vi "AccelerationAttemptLEDWinker.vi"(6 "inputError":errorcluster, 8 "StateValue":T1, 9 "CurrentEntry":string, 10 "EventProgressDataInput":string[][](array[string]), 11 "inputRefOfLED":refnum<vi>[](array[refnum])) -> (4 "outputError":errorcluster)   [LabVIEW 2020]
uses:
  Control/AccelerationState.ctl
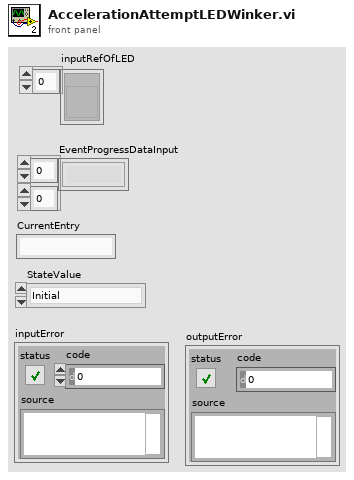
[diagram p1: front panel]
types:
  T1 = typedef "AccelerationState.ctl" = enum16{"Initial", "InputInfomation", "Ready", "Running", "FinshRunning", "LogRecord", "HardwareRelease", "WaittingforNext", "ProgramStop"}
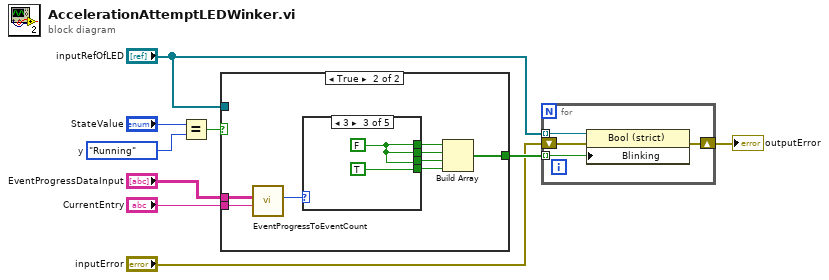
[diagram p0: block diagram]
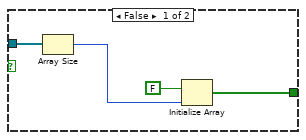
[diagram p2: hidden frame]
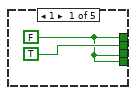
[diagram p3: hidden frame]
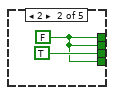
[diagram p4: hidden frame]
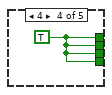
[diagram p5: hidden frame]
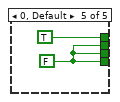
[diagram p6: hidden frame]
diagram:
  w1 = AccelerationState."Running"  # y
  n1 = Equal?(x="StateValue", y=w1) -> (x = y?=w2:bool)
  n2 = case shown="True" w2 {
    tunnel: "EventProgressDataInput" -> [_ w20]
    tunnel: "CurrentEntry" -> [_ w19]
    tunnel: [w9 w18] -> w6
    tunnel: "inputRefOfLED" -> [w12 _]
    frame False {
      n3 = Array Size(array=w12) -> (size(s)=w11:i32)
      n4 = Initialize Array "Initialize Array"(FALSE, w11) -> (w9:bool[])
    }
    frame True {
      n5 = call "EventProgressToEventCount.vi"("CurrentEntry"=w19, "EventProgressDataInput"=w20) -> ("EventCount"=w13:i32)  [unwired: 9 in]
      n6 = case shown="3" w13 {
        tunnel: [w21 w23 w25 w27 TRUE] -> w17
        tunnel: [TRUE w23 w25 w27 w28] -> w16
        tunnel: [w21 TRUE w25 w27 w28] -> w15
        tunnel: [w21 w23 TRUE w27 w28] -> w14
        frame 1 {
          w21 = FALSE
        }
        frame 2 {
          w23 = FALSE
        }
        frame 3 {
          w25 = FALSE
        }
        frame 4 {
          w27 = TRUE
        }
        frame 0, Default {
          w28 = FALSE
        }
      }
      n7 = Build Array "Build Array"(w17, w16, w15, w14) -> (w18:bool[])
    }
  }
  n8 = for {
    shift-right: [w32] -> _
    shift-left: _ -> [w33]
    tunnel: w6 -> [w31] mode=indexing
    tunnel: "inputRefOfLED" -> [w30] mode=indexing
    n9 = property class="Bool (strict)"(reference=w30, error in=w33, "Blinking"=w31) -> (error out=w32:errorcluster)  [unwired: 1 out]
  }
  "outputError" <- "inputError"
